vi "BoolWeightCalc.vi"(6 "Low Weight":dbl=1.0, 7 "High Weight":dbl=1.0, 8 "Reset":bool, 9 "True At 0?":bool=TRUE, 10 "Enable Tracking":bool=TRUE, 11 "Signal In":bool) -> (3 "Signal Out":bool)   [LabVIEW 2016]
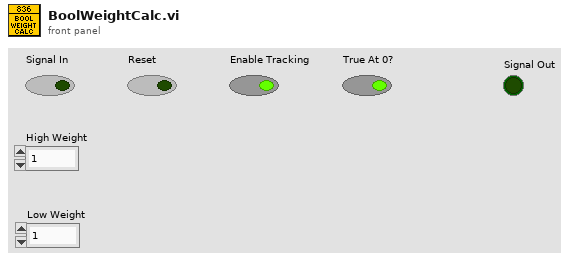
[diagram p1: front panel]
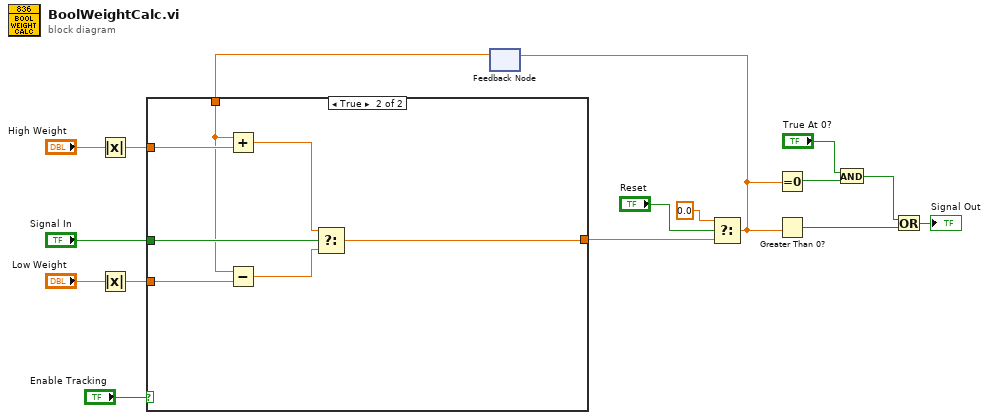
[diagram p0: block diagram]
diagram:
  n1 = Absolute Value(x="High Weight") -> (abs(x)=w2:dbl)
  n2 = Absolute Value(x="Low Weight") -> (abs(x)=w1:dbl)
  n3 = feedback #1() -> (w12:dbl)  [unwired: 1 in]
  n4 = case shown="True" "Enable Tracking" {
    tunnel: [w17 w18] -> w13
    tunnel: w12 -> [w17 w21]
    tunnel: "Signal In" -> [_ w24]
    tunnel: w2 -> [_ w22]
    tunnel: w1 -> [_ w20]
    frame False {
    }
    frame True {
      n5 = Add(x=w21, y=w22) -> (x+y=w23:dbl)
      n6 = Subtract(x=w21, y=w20) -> (x-y=w19:dbl)
      n7 = Select(t=w23, s=w24, f=w19) -> (s? t:f=w18:dbl)
    }
  }
  n8 = Select(t=0.0, s="Reset", f=w13) -> (s? t:f=w11:dbl)
  n9 = feedback-in #1(w11) -> ()
  n10 = Equal To 0?(x=w11) -> (x = 0?=w10:bool)
  n11 = Greater Than 0?(x=w11) -> (x > 0?=w6:bool)
  n12 = And(x="True At 0?", y=w10) -> (x .and. y?=w7:bool)
  n13 = Or(x=w7, y=w6) -> (x .or. y?=→"Signal Out":bool)
